vi "Uim ENA wrapper.vi"(8 "error in (no error)":errorcluster caption="错误输入（无错误）", 9 "bAckEna":i32, 10 "dwCanNodeId":u32, 11 "dwDevIndex":u32) -> (0 "error out":errorcluster caption="错误输出", 1 "BASIC_ACK_OBJ":T1, 3 "function return":u32)   [LabVIEW 2016, in "UISimCanFunc_wrapper.lvlib"]
doc: "_declspec (dllexport) DWORD UimENA_wrapper(DWORD dwDevIndex, DWORD dwCanNodeId, BOOL bAckEna, P_BASIC_ACK_OBJ pBasicAckobj);"
uses:
  <userlib>/UISimCanFunc_wrapper/UISimCanFunc_wrapper.lvlib
  <userlib>/UISimCanFunc_wrapper/ctl/BASIC_ACK_OBJ.ctl
  <userlib>/UISimCanFunc_wrapper/UISimCanFunc_wrapper.dll
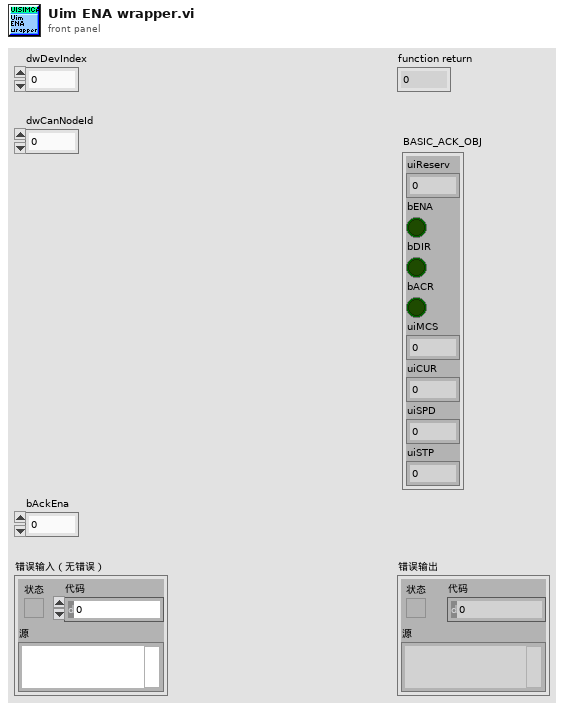
[diagram p1: front panel]
types:
  T1 = typedef "UISimCanFunc_wrapper.lvlib/BASIC_ACK_OBJ.ctl" = cluster{"uiReserv":u32, "bENA":bool, "bDIR":bool, "bACR":bool, "uiMCS":u32, "uiCUR":u32, "uiSPD":u32, "uiSTP":u32}
  T2 = cluster{"uiReserv":u32, "bENA":i32, "bDIR":i32, "bACR":i32, "uiMCS":u32, "uiCUR":u32, "uiSPD":u32, "uiSTP":u32}
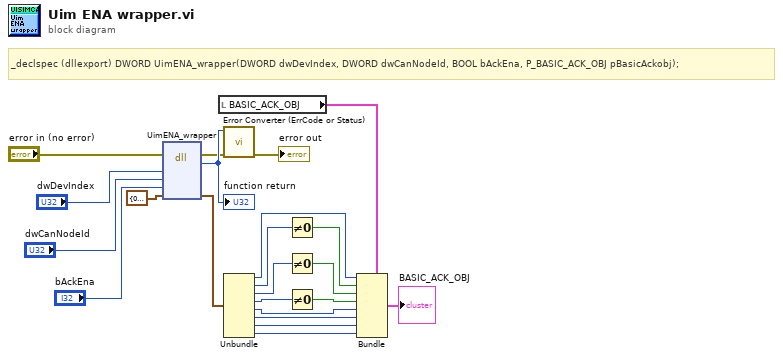
[diagram p0: block diagram]
diagram:
  # "_declspec (dllexport) DWORD UimENA_wrapper(DWORD dwDevIndex, DWORD dwCanNodeId, BOOL bAckEna, P_BASIC_ACK_OBJ pBasicAckobj);"
  n1 = dll-call lib="C:/Program Files (x86)/National Instruments/LabVIEW 2016/user.lib/UISimCanFunc_wrapper/UISimCanFunc_wrapper.*" fn="UimENA_wrapper"(error in="error in (no error)", "dwDevIndex"="dwDevIndex", "dwCanNodeId"="dwCanNodeId", "bAckEna"="bAckEna", "pBasicAckobj"=T2 {"uiReserv"=0, "bENA"=0, "bDIR"=0, "bACR"=0, "uiMCS"=0, "uiCUR"=0, "uiSPD"=0, "uiSTP"=0}) -> (error out=w16:errorcluster, w22:u32, "pBasicAckobj"=w14:T2)  [unwired: 5 in, 1 out]
  "function return" <- w22
  n2 = local read "BASIC_ACK_OBJ"() -> (w13:T1)
  n3 = call <userlib>:"Error Converter (ErrCode or Status).vi"("error in (no error)"=w16, "error code"=w22) -> ("error out"=→"error out":errorcluster)  [unwired: 9 in]
  n4 = Unbundle(w14) -> ("uiReserv"=w12:u32, "bENA"=w11:i32, "bDIR"=w10:i32, "bACR"=w9:i32, "uiMCS"=w5:u32, "uiCUR"=w4:u32, "uiSPD"=w3:u32, "uiSTP"=w2:u32)
  n5 = Not Equal To 0?(x=w11) -> (x != 0?=w8:bool)
  n6 = Not Equal To 0?(x=w10) -> (x != 0?=w7:bool)
  n7 = Not Equal To 0?(x=w9) -> (x != 0?=w6:bool)
  n8 = Bundle(cluster=w13, "uiReserv"=w12, "bENA"=w8, "bDIR"=w7, "bACR"=w6, "uiMCS"=w5, "uiCUR"=w4, "uiSPD"=w3, "uiSTP"=w2) -> (→"BASIC_ACK_OBJ":T1)
